vi "InitPGI.vi"(0 "DeviceNumber":i32=1, 11 "error in (no error)":errorcluster caption="错误输入（无错误）") -> (4 "SENSOR":T1, 15 "error out":errorcluster caption="错误输出")   [LabVIEW 2020]
doc: "该模板用于创建子VI。"
panel:
  out "function return":i32
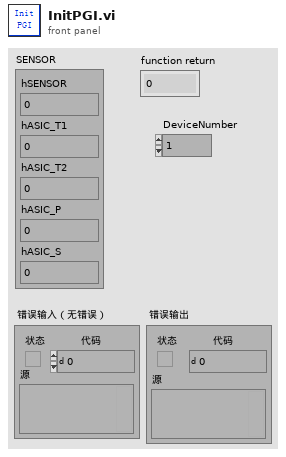
[diagram p1: front panel]
types:
  T1 = cluster{"hSENSOR":i32, "hASIC_T1":i32, "hASIC_T2":i32, "hASIC_P":i32, "hASIC_S":i32}
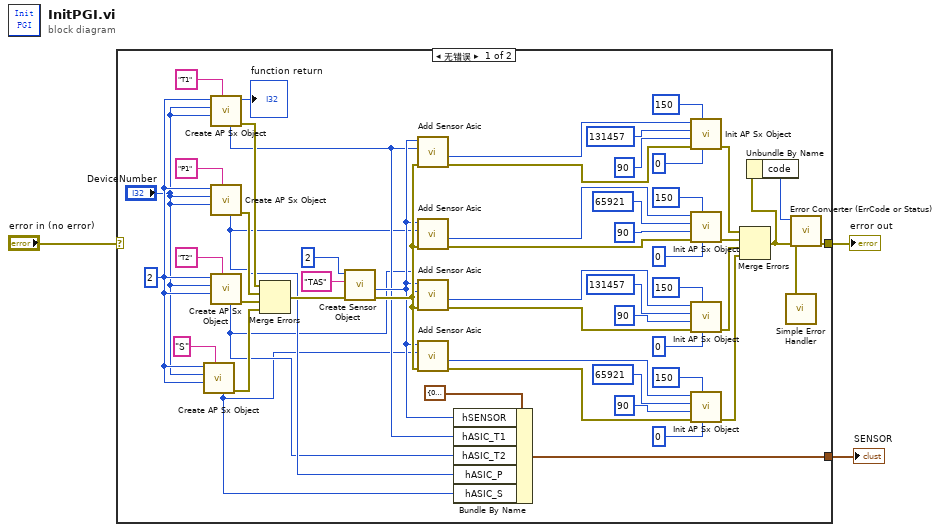
[diagram p0: block diagram]
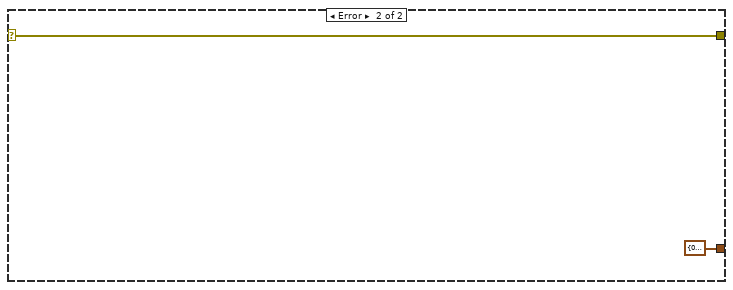
[diagram p2: hidden frame]
diagram:
  n1 = case shown="无错误" "error in (no error)" {
    selector: "error in (no error)" -> [_ w58]
    tunnel: [w6 w58] -> w2
    tunnel: [w9 T1 {"hSENSOR"=0, "hASIC_T1"=0, "hASIC_T2"=0, "hASIC_P"=0, "hASIC_S"=0} ("SENSOR")] -> w1
    frame No Error {
      w54 = 2 ("pgiType")
      n2 = call "Create AP Sx Object.vi"("asicName"="S" ("AsicName"), "pgiChannel"=w54, "pgiDevNum"="DeviceNumber", "pgiType"=w54) -> ("error out"=w55:errorcluster, "asicHandle out"=w10:i32)  [unwired: 4 in, 2 out]
      n3 = call "Create AP Sx Object.vi"("asicName"="T1" ("AsicName"), "pgiChannel"="DeviceNumber", "pgiDevNum"="DeviceNumber", "pgiType"=w54) -> ("error out"=w48:errorcluster, "function return"=→"function return":i32, "asicHandle out"=w13:i32)  [unwired: 4 in, 1 out]
      n4 = call "Create AP Sx Object.vi"("asicName"="P1" ("AsicName"), "pgiChannel"="DeviceNumber", "pgiDevNum"="DeviceNumber", "pgiType"=w54) -> ("error out"=w50:errorcluster, "asicHandle out"=w12:i32)  [unwired: 4 in, 2 out]
      n5 = call "Create AP Sx Object.vi"("asicName"="T2" ("AsicName"), "pgiChannel"=w54, "pgiDevNum"="DeviceNumber", "pgiType"=w54) -> ("error out"=w52:errorcluster, "asicHandle out"=w11:i32)  [unwired: 4 in, 2 out]
      n6 = Merge Errors(w48, w50, w52, w55) -> (w45:errorcluster)
      n7 = call "Create Sensor Object.vi"("error in (no error)"=w45, "sensorName"="TAS" ("SensorName"), "pgiType"=2) -> ("error out"=w44:errorcluster, "sensorHandle out"=w14:i32)  [unwired: 5 in, 2 out]
      n8 = call "Add Sensor Asic.vi"("error in (no error)"=w44, "asicHandle"=w13, "sensorHandle"=w14) -> ("error out"=w43:errorcluster, "AsicHandle out"=w41:i32)  [unwired: 6 in, 1 out]
      n9 = call "Add Sensor Asic.vi"("error in (no error)"=w44, "asicHandle"=w12, "sensorHandle"=w14) -> ("error out"=w32:errorcluster, "AsicHandle out"=w30:i32)  [unwired: 6 in, 1 out]
      n10 = call "Add Sensor Asic.vi"("error in (no error)"=w44, "asicHandle"=w11, "sensorHandle"=w14) -> ("error out"=w25:errorcluster, "AsicHandle out"=w23:i32)  [unwired: 6 in, 1 out]
      n11 = call "Add Sensor Asic.vi"("error in (no error)"=w44, "asicHandle"=w10, "sensorHandle"=w14) -> ("error out"=w18:errorcluster, "AsicHandle out"=w17:i32)  [unwired: 6 in, 1 out]
      n12 = Bundle By Name(cluster=T1 {"hSENSOR"=0, "hASIC_T1"=0, "hASIC_T2"=0, "hASIC_P"=0, "hASIC_S"=0} ("SENSOR"), "hSENSOR"=w14, "hASIC_T1"=w13, "hASIC_T2"=w11, "hASIC_P"=w12, "hASIC_S"=w10) -> (w9:T1)
      n13 = call "Init AP Sx Object.vi"("otpOffset"=0, "otpCurrent"=150, "error in (no error)"=w43, "outCurrent"=90, "asicType"=131457, "asicHandle"=w41) -> ("error out"=w42:errorcluster)  [unwired: 4 in, 1 out]
      n14 = call "Init AP Sx Object.vi"("otpOffset"=0, "otpCurrent"=150, "error in (no error)"=w32, "outCurrent"=90, "asicType"=65921, "asicHandle"=w30) -> ("error out"=w31:errorcluster)  [unwired: 4 in, 1 out]
      n15 = call "Init AP Sx Object.vi"("otpOffset"=0, "otpCurrent"=150, "error in (no error)"=w25, "outCurrent"=90, "asicType"=131457, "asicHandle"=w23) -> ("error out"=w24:errorcluster)  [unwired: 4 in, 1 out]
      n16 = call "Init AP Sx Object.vi"("otpOffset"=0, "otpCurrent"=150, "error in (no error)"=w18, "outCurrent"=90, "asicType"=65921, "asicHandle"=w17) -> ("error out"=w16:errorcluster)  [unwired: 4 in, 1 out]
      n17 = Merge Errors(w42, w31, w24, w16) -> (w5:errorcluster)
      n18 = Unbundle By Name(w5) -> ("code"=w4:i32)
      n19 = call "Error Converter (ErrCode or Status).vi"("error in (no error)"=w5, "error code"=w4) -> ("error out"=w6:errorcluster)  [unwired: 9 in]
      n20 = call <vilib>:"Simple Error Handler.vi"("error in (no error)"=w6) -> ()  [unwired: 4 in, 5 out]
    }
    frame Error {
    }
  }
  "error out" <- w2
  "SENSOR" <- w1
